vi "Initialize Daemon.vi"(8 "error in":errorcluster, 9 "Data Model":refnum<class "Device Data Model.lvclass">, 11 "TCP slave in":refnum<class "TCP Server.lvclass">) -> (0 "error out":errorcluster, 3 "TCP slave out":refnum<class "TCP Server.lvclass">)   [LabVIEW 2021, in "WebSockets.lvlib" / "TCP Server.lvclass"]
doc: "Launches the connection daemon and creates the notifier which will allow it to quit."
uses:
  TCP Server.lvclass
  TCP Server.lvclass/TCP Server.ctl
  TCP Daemon.vi
  Connection.ctl
  Connection Counter.ctl
  WebSocket Server.lvclass
  Modbus_v121c/Data Model/Device Data Model.lvclass
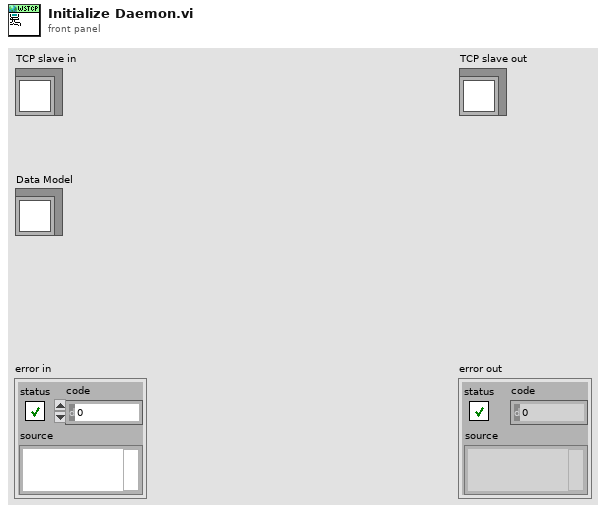
[diagram p1: front panel]
types:
  T1 = typedef "WebSockets.lvlib/TCP Server.lvclass/Connection Counter.ctl" = cluster{"Currently Connected":u32, "Connection Records":refnum<data-value>[]}
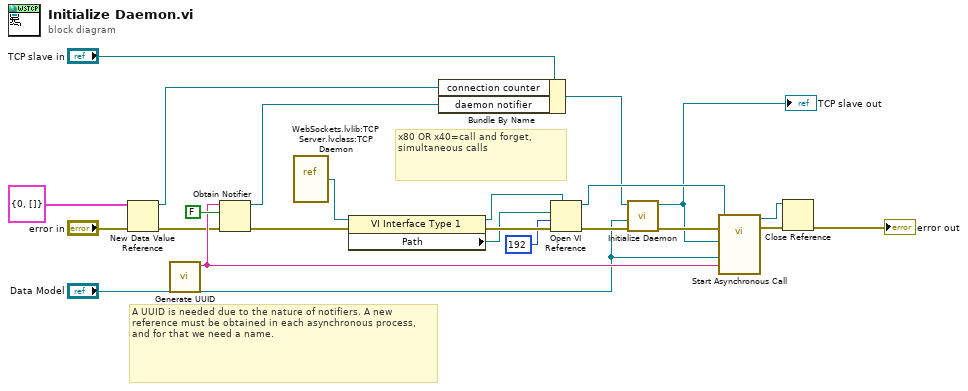
[diagram p0: block diagram]
diagram:
  # "x80 OR x40=call and forget, simultaneous calls"
  # "A UUID is needed due to the nature of notifiers. A new reference must be obtained in each asynchronous process, and for that we need a name."
  n1 = New Data Value Reference(data value=T1 {"Currently Connected"=0, "Connection Records"=[]} ("Connection Counter"), error in="error in") -> (data value reference=w6:refnum<data-value>, error out=w7:errorcluster)
  n2 = call "Generate UUID.vi"() -> ("UUID"=w13:string)  [unwired: 11 in]
  n3 = Obtain Notifier(name (unnamed)=w13, notification data type=FALSE, error in (no error)=w7) -> (notifier out=w14:refnum<notifier>, error out=w16:errorcluster)  [unwired: 1 in, 1 out]
  n4 = vi-ref "WebSockets.lvlib:TCP Server.lvclass:TCP Daemon.vi"() -> (w21:refnum<vi>)
  n5 = property class="VI Interface Type 1"(reference=w21, error in=w16) -> (reference out=w2:refnum<vi>, error out=w20:errorcluster, "Path"=w19:path)
  n6 = Bundle By Name(cluster="TCP slave in", "connection counter"=w6, "daemon notifier"=w14) -> (w11:refnum<class "TCP Server.lvclass">)
  n7 = Open VI Reference(type specifier VI Refnum (for type only)=w2, vi path=w19, options=192 ("x .or. y?"), error in (no error)=w20) -> (vi reference=w18:refnum<vi>, error out=w10:errorcluster)  [unwired: 2 in]
  n8 = call-parent "Initialize Daemon.vi"("error in"=w10, "Device Data Model"="Data Model", "network slave in"=w11) -> ("error out"=w12:errorcluster, "network slave out"=w9:refnum<class "TCP Server.lvclass">)  [unwired: 7 in]
  "TCP slave out" <- w9
  n9 = call-by-ref "Start Asynchronous Call"(reference=w18, error in=w12, "UUID"=w13, "Device Data Model"="Data Model", "TCP slave in"=w9) -> (reference out=w3:refnum<vi>, error out=w22:errorcluster)  [unwired: 9 in]
  n10 = Close Reference(reference=w3, error in (no error)=w22) -> (error out=→"error out":errorcluster)
